vi "Actor Core.vi"(8 "error in":errorcluster, 11 "XY Stage Process in":refnum<class "XY Stage Process.lvclass">) -> (0 "error out":errorcluster, 3 "Actor out":refnum<class "Actor.lvclass">)   [LabVIEW 2022 SP3, in "XY Stage Process.lvlib" / "XY Stage Process.lvclass"]
doc: "(<B>Filename</B>: Actor Framework.lvlib:Actor.lvclass:Actor Core.vi)\n\nReceives messages to the actor, reacts to them, and initiates any error handling that may shut the actor down.\n\nDescendant classes may override this VI to append parallel tasks for the actor to complete while it handles messages. Overrides use the Call Parent Class Method node."
uses:
  XY Stage Process.lvclass
  <vilib>/ActorFramework/Actor/Actor.lvclass
  XY Stage Process.lvclass/XY Stage Process.ctl
  <vilib>/MGI/Monitored Actor/Monitored Actor/Monitored Actor/Monitored Actor.lvclass
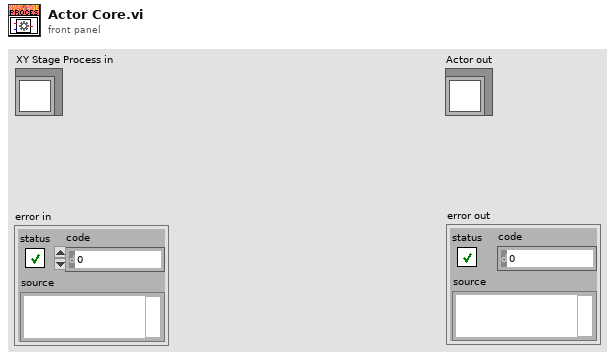
[diagram p1: front panel]
types:
  T1 = typedef "XY Stage Process.lvlib/XY Stage Process.lvclass/Privite Events.ctl" = cluster{"Stop":refnum<user-event>}
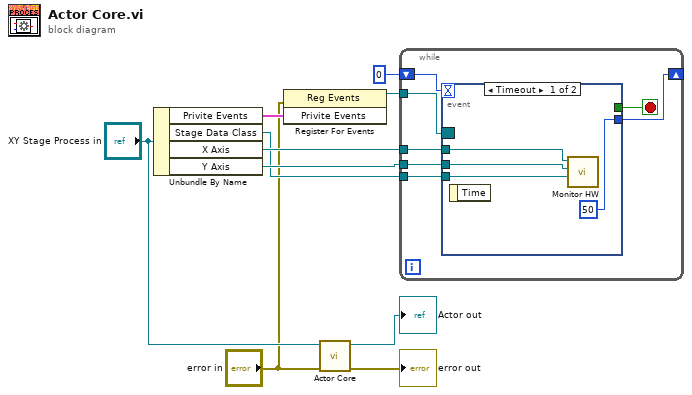
[diagram p0: block diagram]
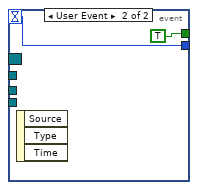
[diagram p2: hidden frame]
diagram:
  n1 = Unbundle By Name("XY Stage Process in") -> ("Privite Events"=w7:T1, "Stage Data Class"=w3:refnum<data-value>, "X Axis"=w5:refnum<class "iMotion Controller.lvclass">, "Y Axis"=w4:refnum<class "iMotion Controller.lvclass">)
  n2 = register-events(error in="error in", w7) -> (reference out=w6:refnum<event-registration>)  [unwired: 1 in, 1 out]
  n3 = call-parent "Actor Core.vi"("error in"="error in", "Actor in"="XY Stage Process in") -> ("error out"=→"error out":errorcluster, "Actor out"=→"Actor out":refnum<class "Actor.lvclass">)  [unwired: 8 in]
  n4 = while {
    tunnel: w6 -> [w17]
    tunnel: w5 -> [w15]
    tunnel: w4 -> [w14]
    tunnel: w3 -> [w13]
    shift-right: [w11] -> _
    shift-left: 0 -> [w12]
    stop <- w16 stop-if-true
    n5 = event shown="[0] Timeout" {
      selector: w17 -> [_ _]
      dyn-events: _ -> [_ _]
      timeout: w12 -> [_ w22]
      tunnel: [_ TRUE] -> w16
      tunnel: w15 -> [w21 _]
      tunnel: w14 -> [w20 _]
      tunnel: w13 -> [w19 _]
      tunnel: [50 w22] -> w11
      event Timeout {
        n6 = event-data() -> ()  [unwired: 1 in, 1 out]
        n7 = call "Monitor HW.vi"("Stage Data Class"=w19, "Y-Axis"=w20, "X Axis"=w21) -> ()  [unwired: 9 in]
      }
      event User Event {
        n8 = event-data() -> ()  [unwired: 1 in, 3 out]
      }
    }
  }
